vi "atomNb.vi"() -> ()   [LabVIEW 2019]
panel:
  out "BG":picture
  out "No MOT":picture
  out "MOT":picture
  in  "cropsize":i16
  in  "cropy":i16
  in  "cropx":i16
  in  "Background":path
  in  "No MOT":path
  in  "MOT":path
  out "Result":dbl
  in  "function name":string
  in  "module path":path
  in  "Python version":string
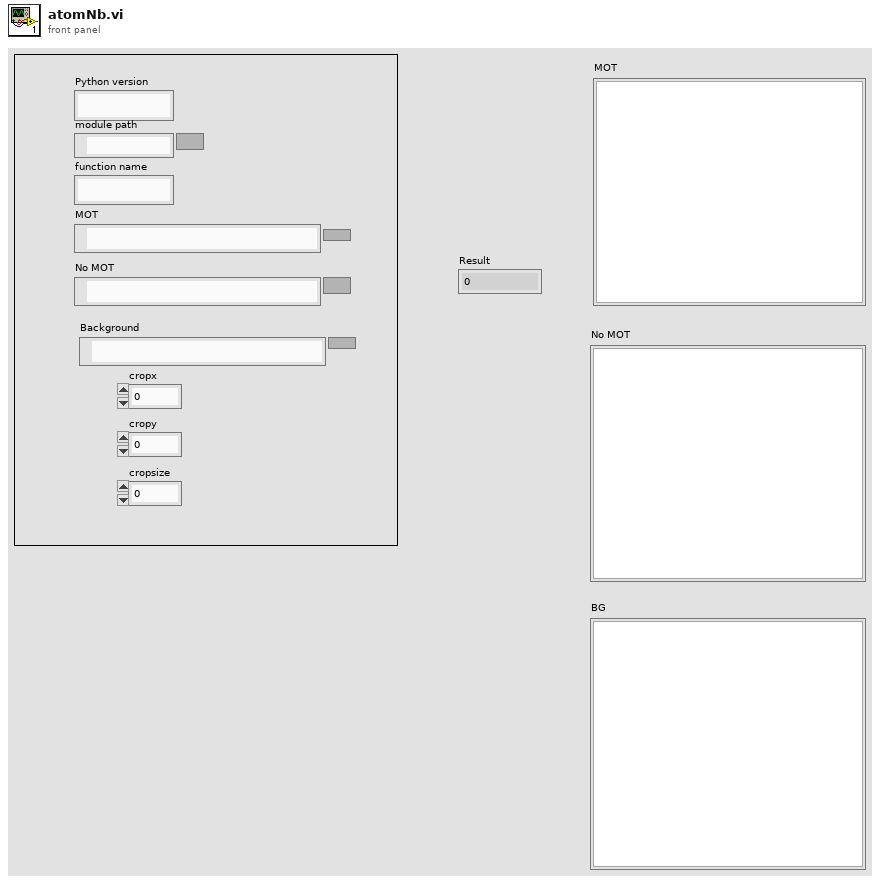
[diagram p1: front panel]
types:
  T1 = typedef "imagedata.ctl" = cluster{"image type":i32, "image depth":i32, "image":u8[], "mask":u8[], "colors":u32[], "Rectangle":cluster{"left":i16, "top":i16, "right":i16, "bottom":i16}}
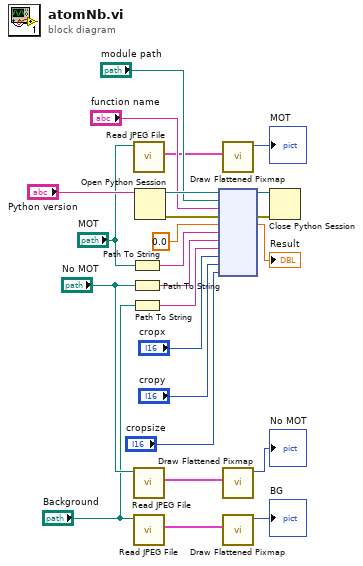
[diagram p0: block diagram]
diagram:
  n1 = Path To String(path="MOT") -> (string=w16:string)
  n2 = Path To String(path="No MOT") -> (string=w15:string)
  n3 = Path To String(path="Background") -> (string=w14:string)
  n4 = call <vilib>:"Read JPEG File.vi"("path to JPEG file"="MOT") -> ("image data"=w8:T1)  [unwired: 8 in, 2 out]
  n5 = call <vilib>:"Read JPEG File.vi"("path to JPEG file"="No MOT") -> ("image data"=w6:T1)  [unwired: 8 in, 2 out]
  n6 = call <vilib>:"Read JPEG File.vi"("path to JPEG file"="Background") -> ("image data"=w4:T1)  [unwired: 8 in, 2 out]
  n7 = Open Python Session(python version="Python version") -> (session out=w22:refnum<k35>, error out=w23:errorcluster)  [unwired: 2 in]
  n8 = node(w22, "module path", "function name", w23, 0.0, w16, w15, w14, "cropx", "cropy", "cropsize") -> (w21:refnum<k35>, w20:errorcluster, →"Result":dbl)  [unwired: 6 in, 2 out]
  n9 = call <vilib>:"Draw Flattened Pixmap.vi"("image data"=w8) -> ("new picture"=→"MOT":picture)  [unwired: 8 in]
  n10 = call <vilib>:"Draw Flattened Pixmap.vi"("image data"=w6) -> ("new picture"=→"No MOT":picture)  [unwired: 8 in]
  n11 = call <vilib>:"Draw Flattened Pixmap.vi"("image data"=w4) -> ("new picture"=→"BG":picture)  [unwired: 8 in]
  n12 = Close Python Session(session in=w21, error in=w20) -> ()  [unwired: 1 out]
